vi "Control ETH008 Relay.vi"(9 "On/Off":bool, 10 "Time ON (secs - 100ms min)  \"0\"=ON":dbl, 11 "Relay Number":i32) -> ()   [LabVIEW 2018]
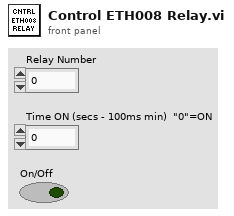
[diagram p1: front panel]
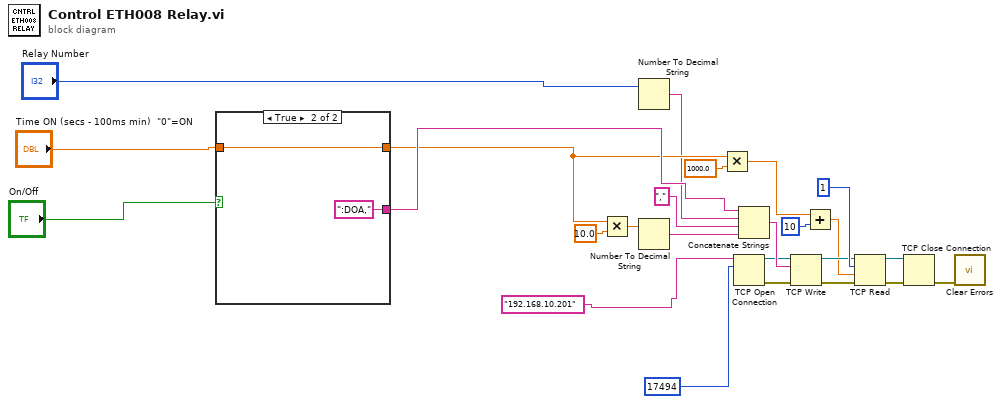
[diagram p0: block diagram]
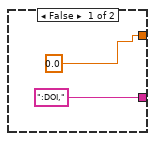
[diagram p2: hidden frame]
diagram:
  n1 = case shown="True" "On/Off" {
    tunnel: "Time ON (secs - 100ms min)  \"0\"=ON" -> [_ w29]
    tunnel: [0.0 w29] -> w23
    tunnel: [":DOI," ("string") ":DOA," ("string")] -> w25
    frame False {
    }
    frame True {
    }
  }
  n2 = Multiply(x=w23, y=10.0) -> (x*y=w18:dbl)
  n3 = Number To Decimal String(number="Relay Number") -> (decimal integer string=w11:string)  [unwired: 1 in]
  n4 = Number To Decimal String(number=w18) -> (decimal integer string=w14:string)  [unwired: 1 in]
  n5 = Multiply(x=w23, y=1000.0) -> (x*y=w20:dbl)
  n6 = TCP Open Connection(address="192.168.10.201", remote port or service name=u16 17494) -> (connection ID=w4:refnum<k5>, error out=w9:errorcluster)  [unwired: 3 in]
  n7 = Concatenate Strings(w25, w11, "," ("string"), w14) -> (w15:string)
  n8 = TCP Write(connection ID=w4, data in=w15, error in (no error)=w9) -> (connection ID out=w5:refnum<k5>, error out=w8:errorcluster)  [unwired: 1 in, 1 out]
  n9 = Add(x=w20, y=10) -> (x+y=w1:dbl)
  n10 = TCP Read(connection ID=w5, bytes to read=1, error in (no error)=w8, 9:w1) -> (connection ID out=w6:refnum<k5>, error out=w7:errorcluster)  [unwired: 1 in, 1 out]
  n11 = TCP Close Connection(connection ID=w6, error in (no error)=w7) -> (error out=w21:errorcluster)  [unwired: 1 in, 1 out]
  n12 = call <vilib>:"Clear Errors.vi"("error in (no error)"=w21) -> ()  [unwired: 5 in, 2 out]
